vi "SimulatedFGA_Lidar.vi"(8 "error in":errorcluster, 9 "initialized \nsonar ray\narray":i32[](array[numeric]), 10 "MDF Image":T1, 11 "RobotPosition":cluster{"xsub":dbl, "ysub":dbl, "heading":dbl}) -> (0 "error out":errorcluster, 3 "LIDAR Data (r:pixel b:degrees)":cluster{"Range":dbl, "Bearing":dbl}[](array[cluster]))   [LabVIEW 2010]
doc: "This SubVI runs a LIDAR simulation at the Forebrain level and pipes the simulated data down to the Hindbrain \"What is around me?\" level. It runs at the Forebrain Level because the IMAQ vis used do not curretnly run at the FPGA level."
uses:
  <vilib>/vision/Image Controls.llb/IMAQ Image.ctl
panel:
  # "This subVI simulated the LIDAR \nat teh Forebrain Level and sends it to \nthe FPGA for insertion into the \ncontrol system at the Hindbrain level the\nactual LIDAR would enter at"
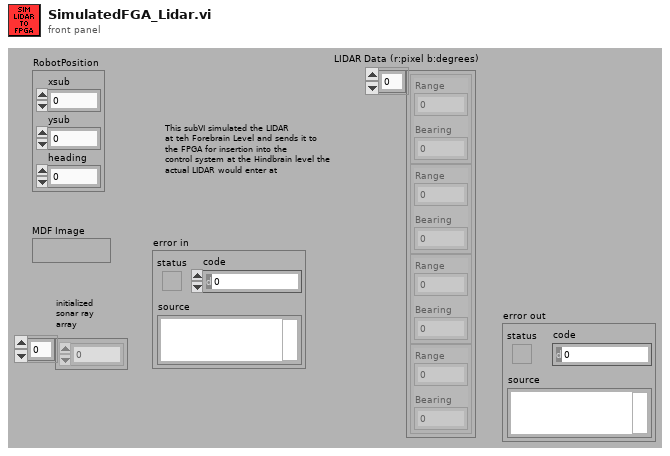
[diagram p1: front panel]
types:
  T1 = typedef "IMAQ Image.ctl" = refnum<image>
  T2 = cluster{"NumberOfBeams":i32, "SonarRange":dbl, "Noise (0.1 to 1)":dbl}
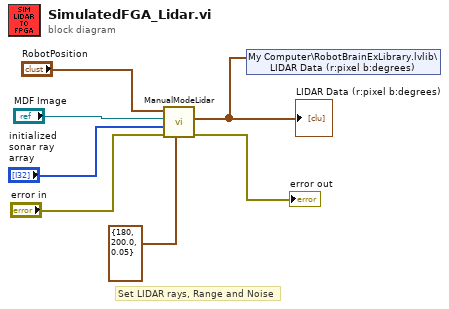
[diagram p0: block diagram]
diagram:
  # "Set LIDAR rays, Range and Noise"
  n1 = call "ManualModeLidar.vi"("LIDARControl"=T2 {"NumberOfBeams"=180, "SonarRange"=200.0, "Noise (0.1 to 1)"=0.05}, "error in"="error in", "initialized \nsonar ray\narray"="initialized \nsonar ray\narray", "MDF Image"="MDF Image", "SubPosition"="RobotPosition") -> ("error out"=→"error out":errorcluster, "LIDAR Data (r:pixel b:degrees)"=w7:cluster{"Range":dbl, "Bearing":dbl}[])  [unwired: 1 in, 2 out]
  "LIDAR Data (r:pixel b:degrees)" <- w7
  n2 = shared-variable "My Computer\\RobotBrainExLibrary.lvlib\\LIDAR Data (r:pixel b:degrees)"(w7) -> ()  [unwired: 1 in, 1 out]
